vi "outstring.vi"(6 "ItemNames 3":string[](array[string]), 7 "ItemNames 2":string[](array[string]), 9 "ItemNames 4":string[](array[string]), 10 "ItemNames":string[](array[string]), 11 "ItemNames 5":string[](array[string])) -> (2 "数组":string[](array[string]), 3 "数组 2":string[][](array[string]))   [LabVIEW 2018]
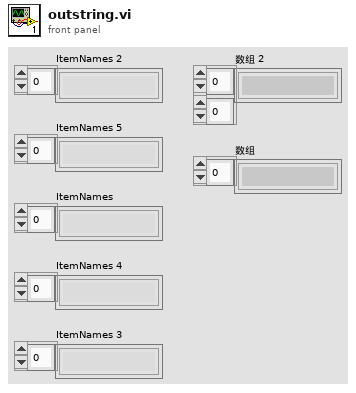
[diagram p1: front panel]
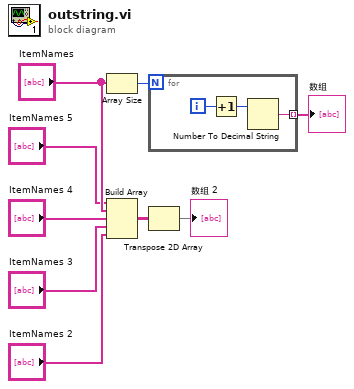
[diagram p0: block diagram]
diagram:
  n1 = Array Size(array="ItemNames") -> (size(s)=w8:i32)
  n2 = Build Array("ItemNames 5", "ItemNames", "ItemNames 4", "ItemNames 3", "ItemNames 2") -> (w5:string[][])
  n3 = for {
    N: w8 -> [_]
    tunnel: [w10] -> w9 mode=indexing
    i -> [w12]
    n4 = Increment(x=w12) -> (x+1=w11:i32)
    n5 = Number To Decimal String(number=w11) -> (decimal integer string=w10:string)  [unwired: 1 out]
  }
  "数组" <- w9
  n6 = Transpose 2D Array(2D array=w5) -> (transposed array=→"数组 2":string[][])
